vi "Configure Hardware.vi"(8 "error in (no error)":errorcluster, 11 "Hardware Resources in":T1) -> (0 "error out":errorcluster, 3 "Hardware Resources out":T1)   [LabVIEW 2017, in "Acquisition.lvlib"]
doc: "Configure the hardware."
uses:
  Acquisition.lvlib
  Hardware Configuration.ctl
  <vilib>/DAQmx/create/channels.llb/DAQmx Create Channel (AI-Voltage-Basic).vi
  <vilib>/DAQmx/configure/timing.llb/DAQmx Timing (Sample Clock).vi
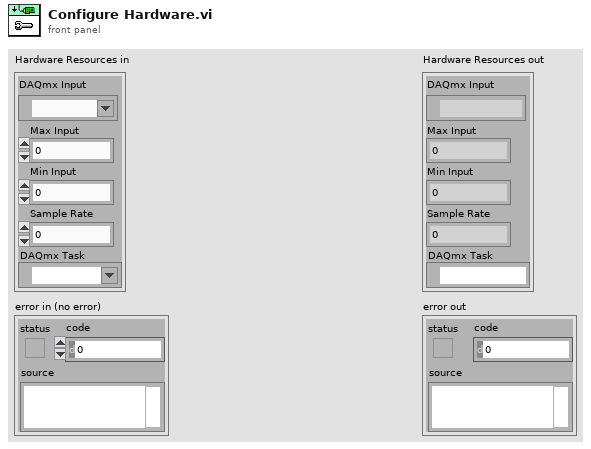
[diagram p1: front panel]
types:
  T1 = typedef "Acquisition.lvlib/Hardware Configuration.ctl" = cluster{"DAQmx Input":tag, "Max Input":dbl, "Min Input":dbl, "Sample Rate":dbl, "DAQmx Task":refnum<k21>}
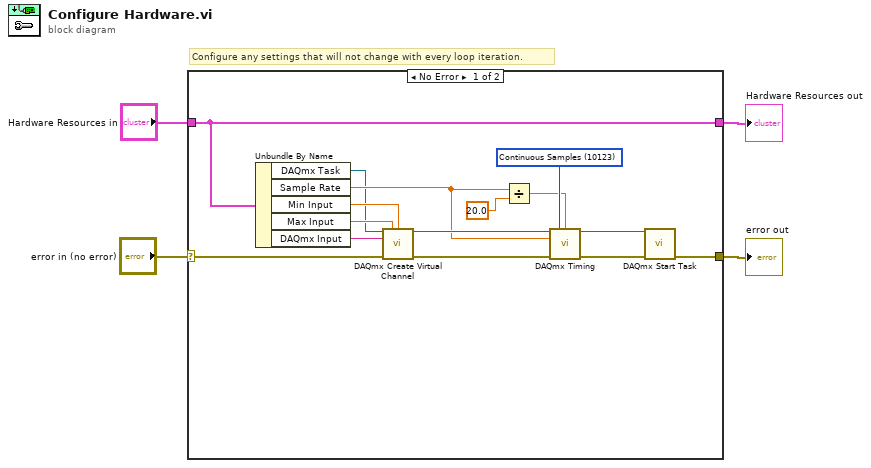
[diagram p0: block diagram]
diagram:
  # "Configure any settings that will not change with every loop iteration."
  n1 = case shown="No Error" "error in (no error)" {
    selector: "error in (no error)" -> [w14 w20]
    tunnel: [w8 w20] -> w3
    tunnel: "Hardware Resources in" -> [w13 w21]
    tunnel: [w13 w21] -> w1
    frame No Error {
      w12 = 10123 items=["Finite Samples"=10178, "Continuous Samples"=10123, "Hardware Timed Single Point"=12522] ("sample mode")
      n2 = Unbundle By Name(w13) -> ("DAQmx Task"=w6:refnum<k21>, "Sample Rate"=w11:dbl, "Min Input"=w17:dbl, "Max Input"=w18:dbl, "DAQmx Input"=w19:tag)
      n3 = call-poly <vilib>:"DAQmx Create Virtual Channel.vi"("task in"=w6, "maximum value"=w18, "minimum value"=w17, "physical channels"=w19, "error in"=w14) -> ("task out"=w16:refnum<k21>, "error out"=w15:errorcluster)  [unwired: 9 in]
      n4 = Divide(x=w11, y=20.0) -> (x/y=w5:dbl)
      n5 = call-poly <vilib>:"DAQmx Timing.vi"("task/channels in"=w16, "sample mode"=w12, "samples per channel"=w5, "rate"=w11, "error in"=w15) -> ("task out"=w9:refnum<k21>, "error out"=w10:errorcluster)  [unwired: 9 in]
      n6 = call <vilib>:"DAQmx Start Task.vi"("task/channels in"=w9, "error in"=w10) -> ("error out"=w8:errorcluster)  [unwired: 12 in, 1 out]
    }
    frame Error {
    }
  }
  "Hardware Resources out" <- w1
  "error out" <- w3
